vi "Test Launcher.vi"   [LabVIEW 2015]
uses:
  Actors/RDS Root Actor/RDS Root Actor/RDS Root Actor.lvclass
  <vilib>/ActorFramework/Actor/Actor.lvclass
panel:
  # "LAUNCHER"
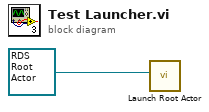
[diagram p0: block diagram]
diagram:
  n1 = call <vilib>:"Launch Root Actor.vi"("Actor"=refnum<class "RDS Root Actor.lvclass"> refnum ("RDS Root Actor.lvlib:RDS Root Actor.lvclass")) -> ()  [unwired: 9 in, 2 out]
